vi "Quantum Composers 9000 Series Recall-Save Configuration.vi"() -> ()   [LabVIEW 2012]
doc: "This VI is an example of how to use subVIs from the QC 9000 series driver to programmatically recall/save a configuration from/to the unit's non-volatile memory.\n\n\nNotes:\n1) The pulse generator keypad is returned to \"Local\" mode when this VI terminates in order to restore manual control to the user.\n2) VISA Version 3.3 or higher must be installed to use this instrument driver."
uses:
  QuantCompControl.llb/Channel Parameters.ctl
  QuantCompControl.llb/System Parameters.ctl
panel:
  in  "Write data \n(off reads data)":bool
  in  "Memory  (1)":i32=1
  in  "System Parameters":T1={"Sys Period"=0.000142, "Sys Mode"=enum."Normal", "Sys Burst #"=4, "Sys DC On"=3, "Sys DC Off"=2, "Sys State"=TRUE, "Sys Gate"=FALSE, "Sys Trig Edge"=TRUE, "Sys Ext Mode"=enum."Disabled", "Sys Trig Lev"=2.5, "Sys Gate Lev "=0.0, "Sys Gate Mode"=enum."Disabled"} {"Sys Gate Lev" format="%.4p"; "Sys Trig Lev" format="%.4p"; "Sys Period" format="%.6p"}
  in  "VISA resource":refnum<visa-resource-name>="TCPIP0::192.168.0.136::2101::SOCKET"
  in  "Channel Parameters":T2[](array[typedef])=[{"Channel"=1, "Chan State"=TRUE, "Chan Sync Source"=0, "Chan Gate Logic"=enum."Disabled", "Chan Mode"=enum."Normal", "Chan Wait #"=0, "Chan Delay"=2e-07, "Chan Width"=1e-06, "Chan Burst #"=5, "Chan DC On"=4, "Chan DC Off"=3, "Chan Polarity"=FALSE, "Chan MUX Value"=1, "Chan Level Out"=enum."TTL", "Chan Lev Adjust"=9.0, "Chan Gate Mode"=enum."Disabled"}, {"Channel"=2, "Chan State"=TRUE, "Chan Sync Source"=0, "Chan Gate Logic"=enum."Disabled", "Chan Mode"=enum."Normal", "Chan Wait #"=0, "Chan Delay"=1.5e-06, "Chan Width"=1e-06, "Chan Burst #"=5, "Chan DC On"=4, "Chan DC Off"=3, "Chan Polarity"=FALSE, "Chan MUX Value"=2, "Chan Level Out"=enum."TTL", "Chan Lev Adjust"=5.0, "Chan Gate Mode"=enum."Disabled"}, {"Channel"=3, "Chan State"=TRUE, "Chan Sync Source"=0, "Chan Gate Logic"=enum."Disabled", "Chan Mode"=enum."Duty Cycle", "Chan Wait #"=0, "Chan Delay"=2e-07, "Chan Width"=0.00994, "Chan Burst #"=5, "Chan DC On"=1, "Chan DC Off"=139, "Chan Polarity"=FALSE, "Chan MUX Value"=4, "Chan Level Out"=enum."TTL", "Chan Lev Adjust"=5.0, "Chan Gate Mode"=enum."Disabled"}, {"Channel"=4, "Chan State"=TRUE, "Chan Sync Source"=0, "Chan Gate Logic"=enum."Disabled", "Chan Mode"=enum."Duty Cycle", "Chan Wait #"=0, "Chan Delay"=2e-07, "Chan Width"=0.00994, "Chan Burst #"=5, "Chan DC On"=1, "Chan DC Off"=139, "Chan Polarity"=FALSE, "Chan MUX Value"=8, "Chan Level Out"=enum."TTL", "Chan Lev Adjust"=5.0, "Chan Gate Mode"=enum."Disabled"}, {"Channel"=1, "Chan State"=TRUE, "Chan Sync Source"=0, "Chan Gate Logic"=enum."Disabled", "Chan Mode"=enum."Duty Cycle", "Chan Wait #"=70, "Chan Delay"=2e-07, "Chan Width"=0.00994, "Chan Burst #"=5, "Chan DC On"=1, "Chan DC Off"=139, "Chan Polarity"=FALSE, "Chan MUX Value"=16, "Chan Level Out"=enum."Adjustable", "Chan Lev Adjust"=9.0, "Chan Gate Mode"=enum."Disabled"}, {"Channel"=6, "Chan State"=TRUE, "Chan Sync Source"=0, "Chan Gate Logic"=enum."Disabled", "Chan Mode"=enum."Duty Cycle", "Chan Wait #"=0, "Chan Delay"=0.0, "Chan Width"=1.2e-06, "Chan Burst #"=5, "Chan DC On"=70, "Chan DC Off"=70, "Chan Polarity"=TRUE, "Chan MUX Value"=32, "Chan Level Out"=enum."TTL", "Chan Lev Adjust"=5.0, "Chan Gate Mode"=enum."Disabled"}, {"Channel"=7, "Chan State"=TRUE, "Chan Sync Source"=0, "Chan Gate Logic"=enum."Disabled", "Chan Mode"=enum."Duty Cycle", "Chan Wait #"=70, "Chan Delay"=0.0, "Chan Width"=1.2e-06, "Chan Burst #"=5, "Chan DC On"=70, "Chan DC Off"=70, "Chan Polarity"=TRUE, "Chan MUX Value"=64, "Chan Level Out"=enum."TTL", "Chan Lev Adjust"=5.0, "Chan Gate Mode"=enum."Disabled"}, {"Channel"=8, "Chan State"=TRUE, "Chan Sync Source"=0, "Chan Gate Logic"=enum."Disabled", "Chan Mode"=enum."Normal", "Chan Wait #"=0, "Chan Delay"=0.0, "Chan Width"=1.6e-06, "Chan Burst #"=5, "Chan DC On"=4, "Chan DC Off"=3, "Chan Polarity"=TRUE, "Chan MUX Value"=128, "Chan Level Out"=enum."TTL", "Chan Lev Adjust"=8.0, "Chan Gate Mode"=enum."Disabled"}] {"Chan Sync Source" items=["System (To)", "Channel A", "Channel B", "Channel C", "Channel D", "Channel E", "Channel F", "Channel G", "Channel H"]; "Chan Width" format="%.3p"; "Chan Delay" format="%.3p"; "Chan Lev Adjust" format="%.3p"; "Channel" items=["Channel A"=1, "Channel B"=2, "Channel C"=3, "Channel D"=4, "Channel E"=5, "Channel F"=6, "Channel G"=7, "Channel H"=8]}
  # "9000 Series\nPulse Generator\nExample Program"
  # "Notes:\n1.  The channel parameters \"Burst #\", \"DC On\", \"DC Off\", and \"Adjustable\" are only updated when operating in the corresponding mode.\n2.  The system parameters  \"Burst #\", \"DC On\", \"DC Off\", and \"Trig Level\"` are only updated when operating in the corresponding mode."
  # "Input"
  # "Triggered"
  # "Gated"
  # "Mode"
  # "Burst"
  # "Duty\nCycle"
  # "Input"
  # "Normal\nSingle\nBurst"
  # "Burst"
  # "Duty Cycle"
  # "Output"
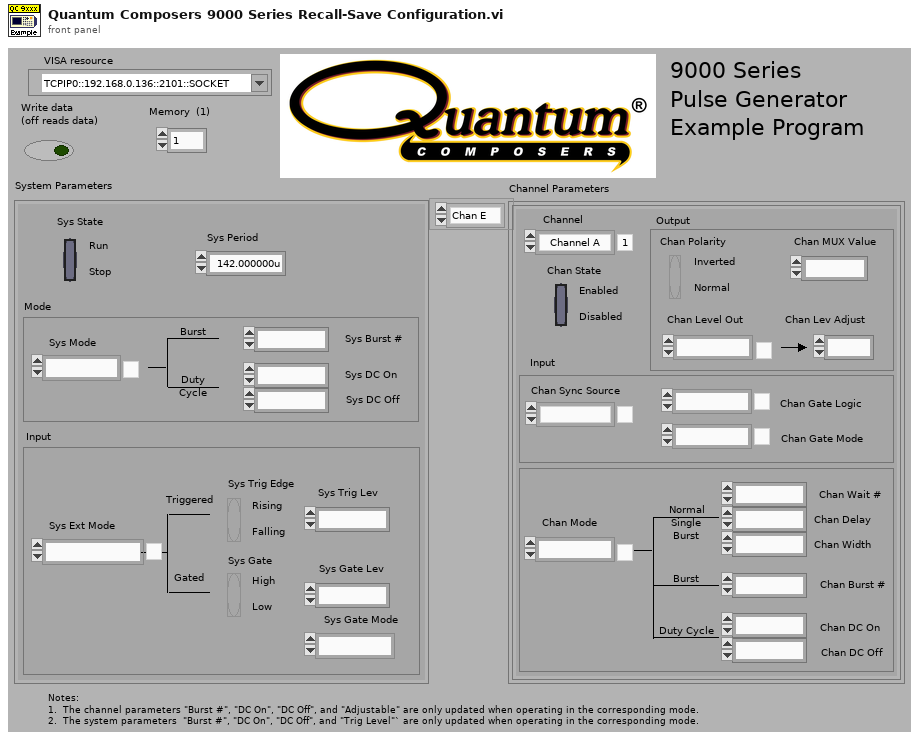
[diagram p1: front panel]
types:
  T1 = typedef "System Parameters.ctl" = cluster{"Sys Period":dbl, "Sys Mode":enum16{"Normal", "Single", "Burst", "Duty Cycle"}, "Sys Burst #":i32, "Sys DC On":i32, "Sys DC Off":i32, "Sys State":bool, "Sys Gate":bool, "Sys Trig Edge":bool, "Sys Ext Mode":enum16{"Disabled", "Triggered", "Gated", "Triggered & Gated"}, "Sys Trig Lev":dbl, "Sys Gate Lev ":dbl, "Sys Gate Mode":enum16{"Disabled", "Pulse Inhibit", "Output Inhibit", "Channel"}}
  T2 = typedef "Channel Parameters.ctl" = cluster{"Channel":i32, "Chan State":bool, "Chan Sync Source":i32, "Chan Gate Logic":enum16{"Disabled", "Low", "High"}, "Chan Mode":enum16{"Normal", "Single", "Burst", "Duty Cycle"}, "Chan Wait #":i32, "Chan Delay":dbl, "Chan Width":dbl, "Chan Burst #":i32, "Chan DC On":i32, "Chan DC Off":i32, "Chan Polarity":bool, "Chan MUX Value":i32, "Chan Level Out":enum16{"TTL", "Adjustable", "35 Volt", "Optical"}, "Chan Lev Adjust":dbl, "Chan Gate Mode":enum16{"Disabled", "Pulse Inhibit", "Output Inhibit"}}
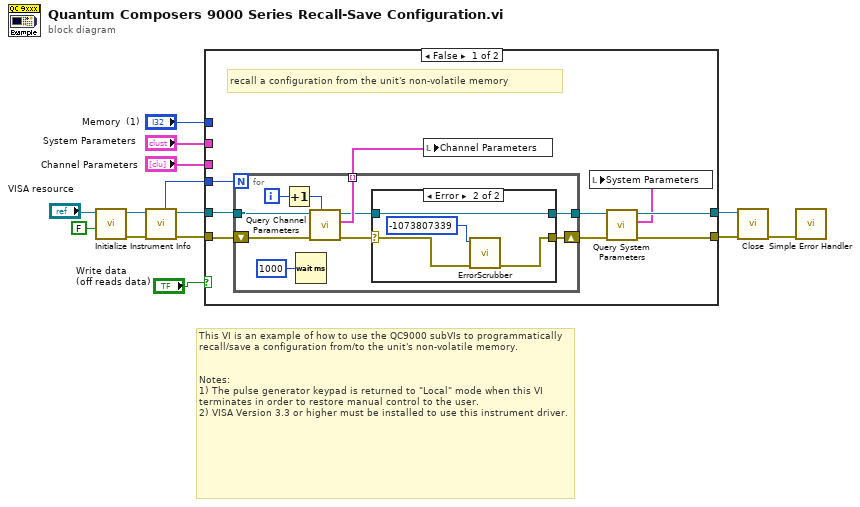
[diagram p0: block diagram]
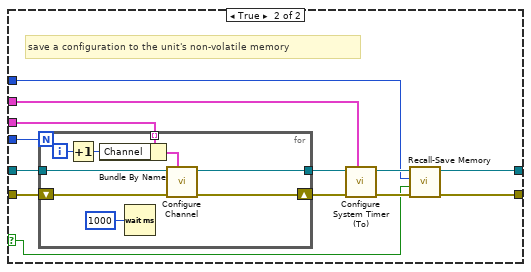
[diagram p3: hidden frame]
diagram:
  # "This VI is an example of how to use the QC9000 subVIs to programmatically recall/save a configuration from/to the unit's non-volatile memory.\n\n\nNotes:\n1) The pulse generator keypad is returned to \"Local\" mode when this VI terminates in order to restore manual control to the user.\n2) VISA Version 3.3 or higher must be installed to use this instrument driver."
  n1 = call "Initialize.vi"("Reset? (T: Yes)"=FALSE, "VISA resource name"="VISA resource") -> ("error out"=w8:errorcluster, "VISA resource name out"=w7:refnum<visa-resource-name>)  [unwired: 3 in, 5 out]
  n2 = call "Instrument Info.vi"("error in (no error)"=w8, "VISA resource name"=w7) -> ("error out"=w4:errorcluster, "VISA resource name out"=w5:refnum<visa-resource-name>, "Channels"=w6:i32)  [unwired: 7 out]
  n3 = case shown="False" "Write data \n(off reads data)" {
    selector: "Write data \n(off reads data)" -> [_ w40]
    tunnel: "Channel Parameters" -> [_ w52]
    tunnel: w5 -> [w16 w51]
    tunnel: w4 -> [w15 w50]
    tunnel: "System Parameters" -> [_ w49]
    tunnel: [w20 w44] -> w11
    tunnel: [w19 w43] -> w10
    tunnel: "Memory  (1)" -> [_ w42]
    tunnel: w6 -> [w17 w41]
    frame False {
      # "recall a configuration from the unit's non-volatile memory"
      n4 = for {
        N: w17 -> [_]
        tunnel: w16 -> [w33]
        tunnel: [w32] -> w23 mode=indexing
        shift-right: [w26] -> w21
        shift-left: w15 -> [w31]
        tunnel: [w24] -> w22
        i -> [w30]
        n5 = Increment(x=w30) -> (x+1=w29:i32)
        n6 = Wait (ms)(milliseconds to wait=u32 1000) -> ()  [unwired: 1 out]
        n7 = call "Query Channel Parameters.vi"("Channel (1:Chan A)"=w29, "error in (no error)"=w31, "VISA resource name"=w33) -> ("error out"=w27:errorcluster, "Chan Parameters"=w32:T2, "VISA resource name out"=w25:refnum<visa-resource-name>)  [unwired: 6 out]
        n8 = case shown="Error" w27 {
          selector: w27 -> [w35 w38]
          tunnel: [w35 w37] -> w26
          tunnel: w25 -> [w34 w39]
          tunnel: [w34 w39] -> w24
          frame No Error {
          }
          frame Error {
            n9 = call "ErrorScrubber.vi"("error in (no error)"=w38, "y"=-1073807339) -> ("error out"=w37:errorcluster)  [unwired: 8 in, 1 out]
          }
        }
      }
      n10 = local write "Channel Parameters"(w23) -> ()
      n11 = call "Query System Parameters.vi"("error in (no error)"=w21, "VISA resource name"=w22) -> ("error out"=w19:errorcluster, "System Parameters"=w18:T1, "VISA resource name out"=w20:refnum<visa-resource-name>)  [unwired: 7 out]
      n12 = local write "System Parameters"(w18) -> ()
    }
    frame True {
      # "save a configuration to the unit's non-volatile memory"
      n13 = for {
        N: w41 -> [_]
        tunnel: [w61] -> w48
        tunnel: w52 -> [w56] mode=indexing
        shift-right: [w60] -> w47
        shift-left: w50 -> [w59]
        tunnel: w51 -> [w58]
        i -> [w55]
        n14 = Increment(x=w55) -> (x+1=w54:i32)
        n15 = Bundle By Name(cluster=w56, "Channel"=w54) -> (w57:T2)
        n16 = Wait (ms)(milliseconds to wait=u32 1000) -> ()  [unwired: 1 out]
        n17 = call "Configure Channel.vi"("Chan Parameters"=w57, "error in (no error)"=w59, "VISA resource name"=w58) -> ("error out"=w60:errorcluster, "VISA resource name out"=w61:refnum<visa-resource-name>)  [unwired: 7 out]
      }
      n18 = call "Configure System Timer (To).vi"("System Parameters"=w49, "error in (no error)"=w47, "VISA resource name"=w48) -> ("error out"=w45:errorcluster, "VISA resource name out"=w46:refnum<visa-resource-name>)  [unwired: 7 out]
      n19 = call "Recall-Save Memory.vi"("error in (no error)"=w45, "Recall/Save (F:Read)"=w40, "Memory  (1)"=w42, "VISA resource name"=w46) -> ("error out"=w43:errorcluster, "VISA resource name out"=w44:refnum<visa-resource-name>)  [unwired: 6 out]
    }
  }
  n20 = call "Close.vi"("error in (no error)"=w10, "VISA resource name"=w11) -> ("error out"=w3:errorcluster)  [unwired: 9 out]
  n21 = call <vilib>:"Simple Error Handler.vi"("error in (no error)"=w3) -> ()  [unwired: 1 in, 8 out]
